vi "Parallel For.vi"() -> ()   [LabVIEW 2014]
panel:
  out "Processing Data":u64(slide) scale=0.0..100000.0
  out "Generating Data":u64(slide) scale=0.0..100000.0
  out "Process":string
  out "Processing Time":dbl
  in  "No. of random generated data":i32
  # "PARALLEL FOR LOOP"
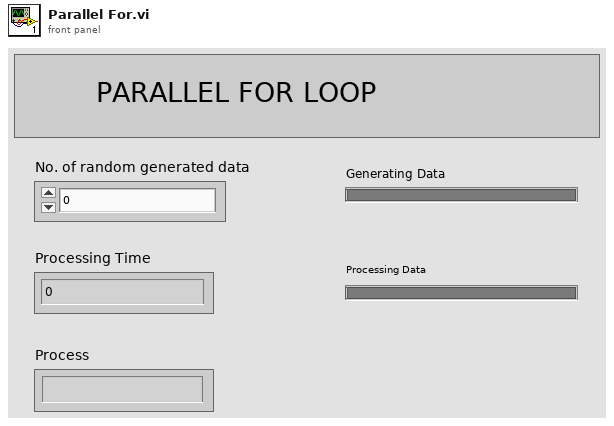
[diagram p1: front panel]
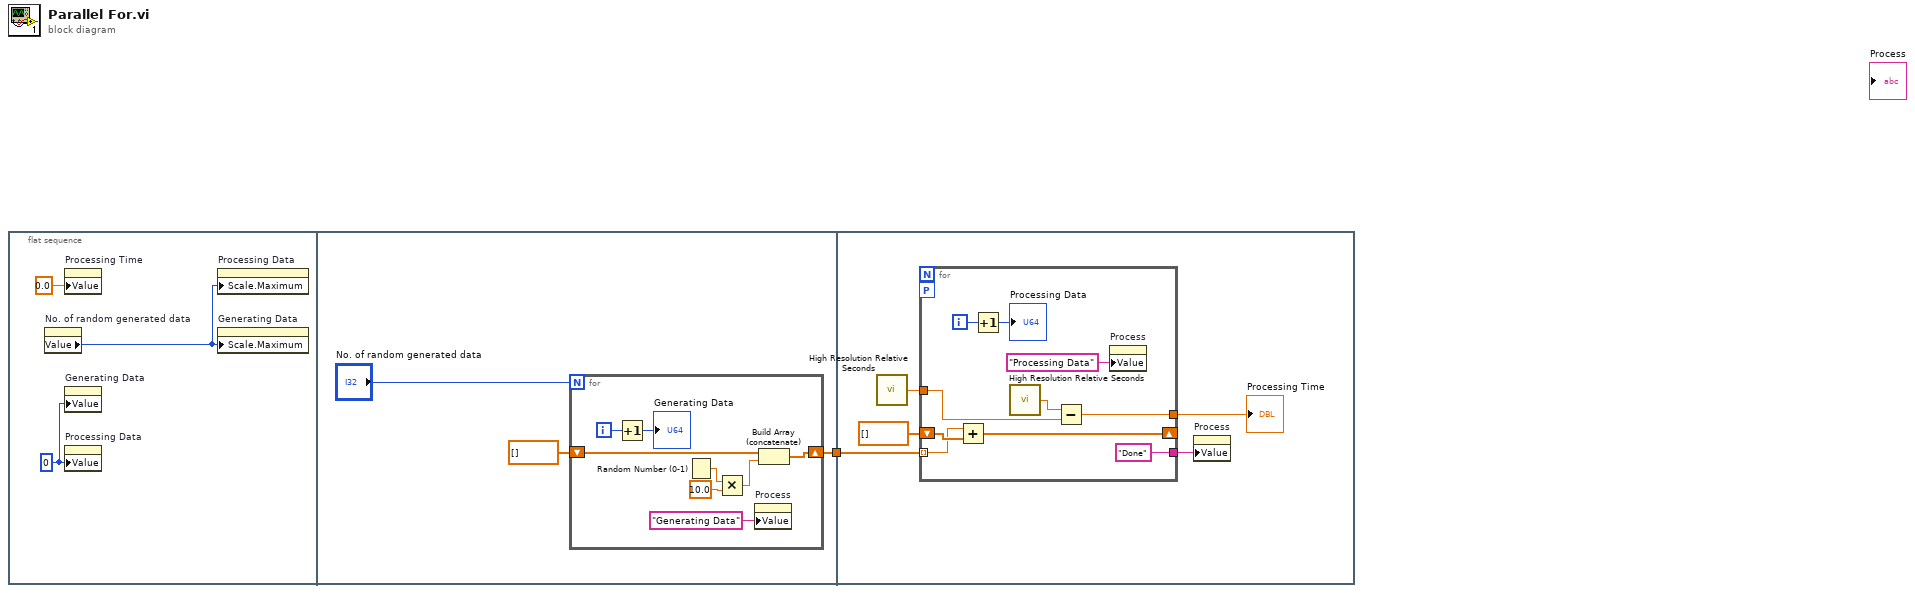
[diagram p0: block diagram]
diagram:
  n1 = flat-sequence {
    tunnel: [w5] -> w1
    tunnel: w1 -> [w16]
    frame #0 {
      w2 = u64 0 ("Generating Data")
      n2 = property on="No. of random generated data" class="DigNum (strict)"() -> ("Value"=w3:i32)  [unwired: 2 in, 2 out]
      n3 = property on="Processing Time" class="DigNum (strict)"("Value"=0.0 ("Processing Time")) -> ()  [unwired: 2 in, 2 out]
      n4 = property on="Generating Data" class="Slide (strict)"("Value"=w2) -> ()  [unwired: 2 in, 2 out]
      n5 = property on="Processing Data" class="Slide (strict)"("Value"=w2) -> ()  [unwired: 2 in, 2 out]
      n6 = property on="Processing Data" class="Slide (strict)"("Scale.Maximum"=w3) -> ()  [unwired: 2 in, 2 out]
      n7 = property on="Generating Data" class="Slide (strict)"("Scale.Maximum"=w3) -> ()  [unwired: 2 in, 2 out]
    }
    frame #1 {
      n8 = for {
        N: "No. of random generated data" -> [_]
        shift-right: [w12] -> w5
        shift-left: dbl[] [] -> [w11]
        i -> [w9]
        n9 = Increment(x=w9) -> (x+1=→"Generating Data":i32)
        n10 = Random Number (0-1)() -> (number: 0 to 1=w15:dbl)
        n11 = Multiply(x=w15, y=10.0) -> (x*y=w13:dbl)
        n12 = property on="Process" class="Str"("Value"="Generating Data") -> ()  [unwired: 2 in, 2 out]
        n13 = Build Array (concatenate)(w11, w13) -> (w12:dbl[])
      }
    }
    frame #2 {
      n14 = call <vilib>:"High Resolution Relative Seconds.vi"() -> ("relative seconds"=w17:dbl)
      n15 = for {
        tunnel: w16 -> [w23] mode=indexing
        tunnel: w17 -> [w29]
        tunnel: [w28] -> w18
        tunnel: ["Done"] -> w19
        shift-right: [w24] -> _
        shift-left: dbl[] [] -> [w25]
        workers-P: _ -> [_]
        i -> [w21]
        n16 = Add(x=w23, y=w25) -> (x+y=w24:dbl[])
        n17 = Increment(x=w21) -> (x+1=→"Processing Data":i32)
        n18 = call <vilib>:"High Resolution Relative Seconds.vi"() -> ("relative seconds"=w30:dbl)
        n19 = Subtract(x=w30, y=w29) -> (x-y=w28:dbl)
        n20 = property on="Process" class="Str"("Value"="Processing Data") -> ()  [unwired: 2 in, 2 out]
      }
      "Processing Time" <- w18
      n21 = property on="Process" class="Str"("Value"=w19) -> ()  [unwired: 2 in, 2 out]
    }
  }
